vi "Write Delay.vi"(8 "error in (no error)":errorcluster, 10 "Delay":dbl, 11 "Output Timer in":refnum<class "Output Timer.lvclass">) -> (0 "error out":errorcluster, 3 "Output Timer out":refnum<class "Output Timer.lvclass">)   [LabVIEW 2012]
uses:
  Output Timer.lvclass
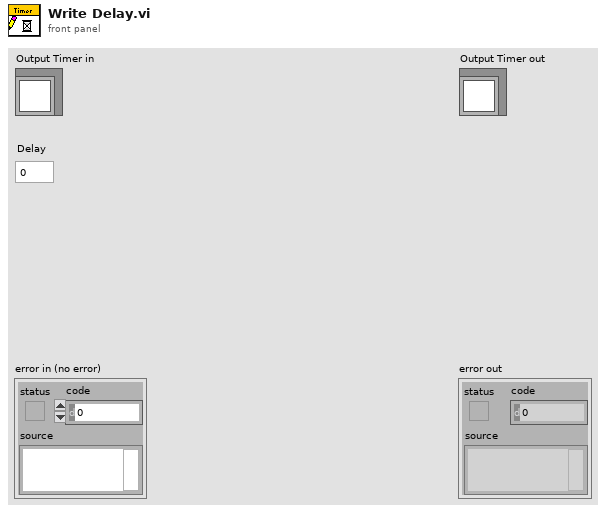
[diagram p1: front panel]
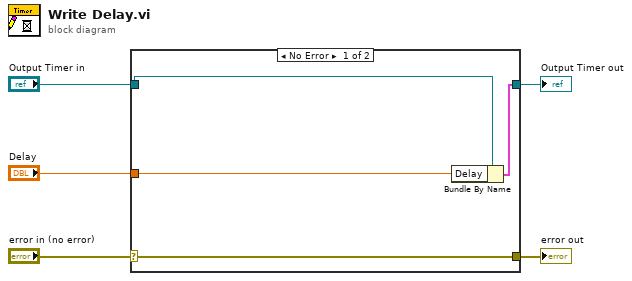
[diagram p0: block diagram]
diagram:
  n1 = case shown="No Error" "error in (no error)" {
    selector: "error in (no error)" -> [w9 w10]
    tunnel: [w9 w10] -> w4
    tunnel: [w6 w11] -> w2
    tunnel: "Output Timer in" -> [w8 w11]
    tunnel: "Delay" -> [w7 _]
    frame No Error {
      n2 = Bundle By Name(cluster=w8, "Delay"=w7) -> (w6:cluster{})
    }
    frame Error {
    }
  }
  "error out" <- w4
  "Output Timer out" <- w2
